vi "GetFunctionArbs.vi"(8 "error in (no error)":errorcluster, 11 "ArbitraryFunction in":refnum<class "ArbitraryFunction.lvclass">) -> (0 "error out":errorcluster, 2 "Arbs":variant, 3 "ArbitraryFunction out":refnum<class "ArbitraryFunction.lvclass">)   [LabVIEW 2018, in "Functions.lvlib" / "ArbitraryFunction.lvclass"]
uses:
  ArbitraryFunction.lvclass
  ArbitraryFunction.lvclass/ArbitraryFunction.ctl
  TypeDefs/Arbs.ctl
  Accessors/Read Arbs.vi
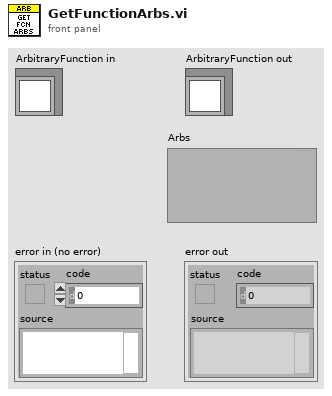
[diagram p1: front panel]
types:
  T1 = typedef "Functions.lvlib/ArbitraryFunction.lvclass/Arbitrary.ctl" = cluster{"Handle":string, "Size":i32, "Gain":dbl, "Offset":dbl, "Waveform":waveform(dbl)}
  T2 = typedef "Functions.lvlib/ArbitraryFunction.lvclass/Arbs.ctl" = cluster{"Handle":string, "Size":i32, "Gain":dbl, "Offset":dbl}
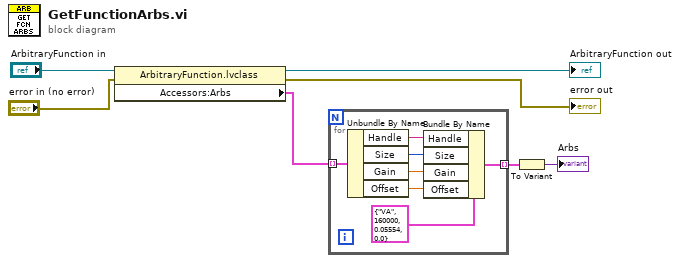
[diagram p0: block diagram]
diagram:
  n1 = property class="ArbitraryFunction.lvclass"(reference="ArbitraryFunction in", error in="error in (no error)") -> (reference out=→"ArbitraryFunction out":refnum<class "ArbitraryFunction.lvclass">, error out=→"error out":errorcluster, "Accessors:Arbs"=w5:T1[])
  n2 = for {
    tunnel: w5 -> [w14] mode=indexing
    tunnel: [w8] -> w4 mode=indexing
    n3 = Unbundle By Name(w14) -> ("Handle"=w12:string, "Size"=w11:i32, "Gain"=w10:dbl, "Offset"=w9:dbl)
    n4 = Bundle By Name(cluster=T2 {"Handle"="VA", "Size"=160000, "Gain"=0.05554, "Offset"=0.0} ("Arbs"), "Handle"=w12, "Size"=w11, "Gain"=w10, "Offset"=w9) -> (w8:T2)
  }
  n5 = To Variant(anything=w4) -> (Variant=→"Arbs":variant)
